vi "uTransport_Destroy.vi"(8 "error in (no error)":errorcluster, 11 "uTransport_uActor in":refnum<class "uTransport_uActor.lvclass">) -> (0 "error out":errorcluster)   [LabVIEW 2023, in "uLib.lvlib" / "uTransport_uActor.lvclass"]
doc: "Invoking this method on an actor does not immediately destroy it, instead it enqueues a self-stop message that takes its turn in the actor's internal FIFO queue.\n\nThis method executes regardless of the error-in state."
uses:
  uTransport_uActor.lvclass
  uMsg/uMsg/uMsg.lvclass/uMsg.ctl
  uTransport_uActor.lvclass/uTransport_uActor.ctl
  uActor/uActor/uActor_CMDs_Prefix.vi
  uActor/uActor/uActor_SimpleSend.vi
  uActor/uActor/uActor_SendMsg.vi
  uMsg/uMsg/uMsg Create.vi
  uTransport_uActor_SendMsg.vi
  uMsg/uMsg/uMsg Update Timestamp.vi
  uData/uData/uData.lvclass
  uTransport/uTransport.lvclass
  uMsg/uMsg/uMsg.lvclass
  uActor/uActor/uActor.lvclass
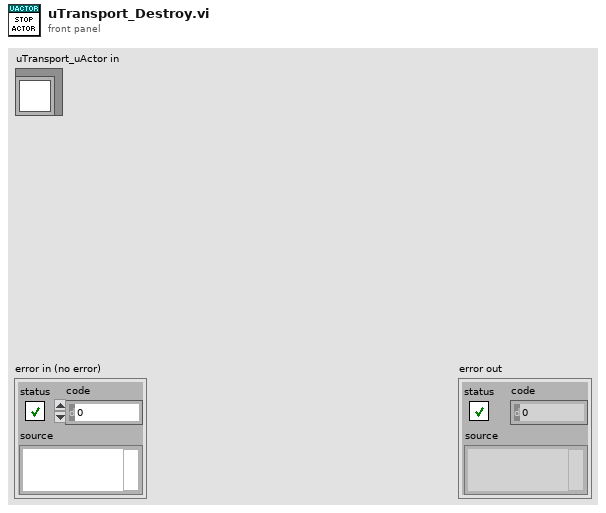
[diagram p1: front panel]
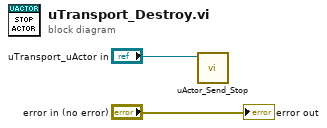
[diagram p0: block diagram]
diagram:
  n1 = call "uActor_Send_Stop.vi"("uActor Transport"="uTransport_uActor in") -> ()  [unwired: 10 in, 1 out]
  "error out" <- "error in (no error)"
